vi "wathc for sweep files.vi"() -> ()   [LabVIEW 2010]
uses:
  watch for sweep file.ctl
panel:
  in  "watch for sweep files in":T1={"file path"=path "C:/data/RUS/Experiment/ProbeTest/systemtest/sweep1", "Watch for sweep files?"=FALSE}
  out "cursor position":dbl=-1.0
  out "history length (min)":dbl=20.0
  out "sweep files in the folder":i32=-1
  out "seconds":i32=189
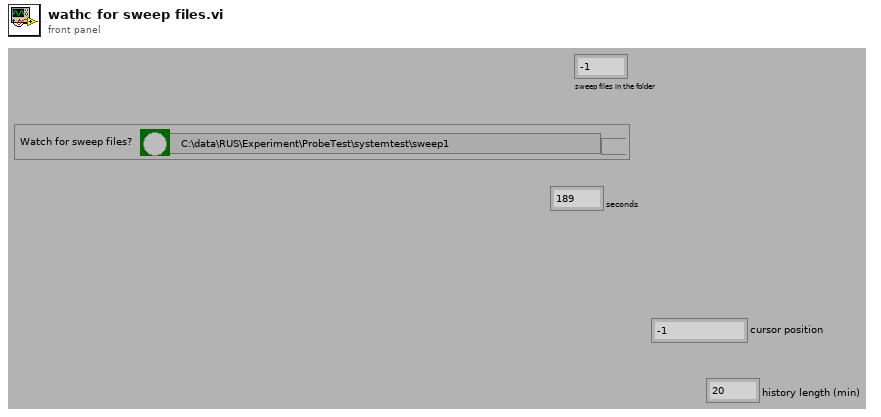
[diagram p1: front panel]
types:
  T1 = typedef "watch for sweep file.ctl" = cluster{"file path":path, "Watch for sweep files?":bool}
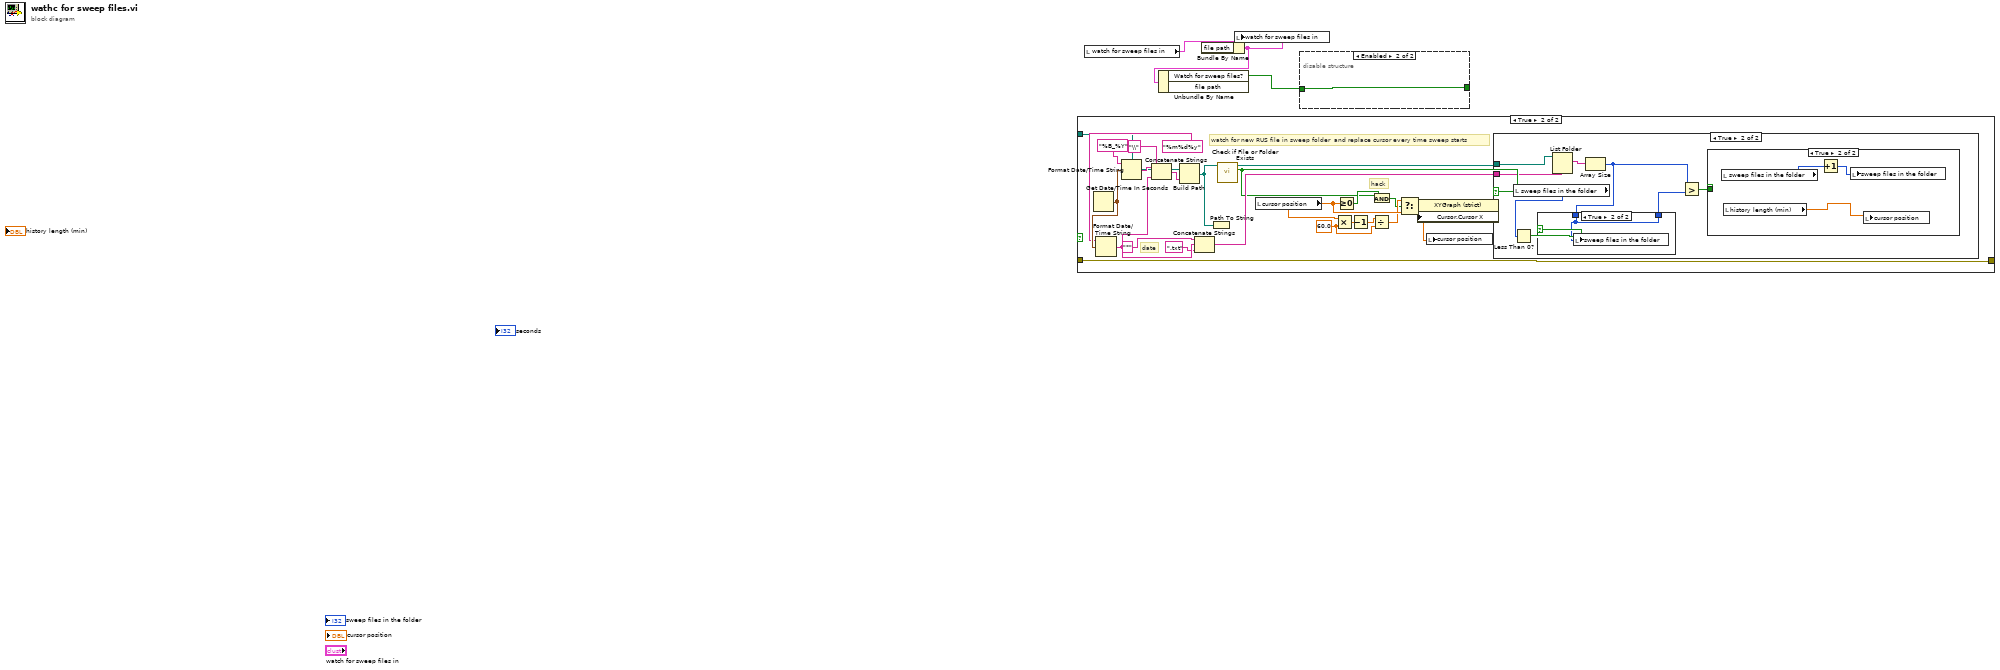
[diagram p0: block diagram]
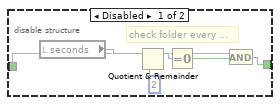
[diagram p2: hidden frame]
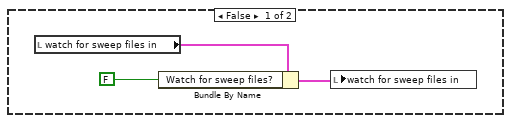
[diagram p4: hidden frame]
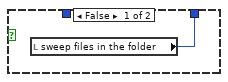
[diagram p6: hidden frame]
diagram:
  n1 = case shown="True" w5 {
    tunnel: [_ w18] -> w2
    tunnel: _ -> [w7 w8]
    tunnel: [w7 w8] -> _
    frame False {
    }
    frame True {
      w17 = 60.0 ("y")
      # "hack"
      # "watch for new RUS file in sweep folder  and replace cursor every time sweep starts"
      # "date"
      n2 = Get Date/Time In Seconds() -> (seconds since 1Jan1904=w27:timestamp)
      n3 = Format Date/Time String(time format string (%c)="%m%d%y", seconds (now)=w27) -> (date/time string=w23:string)  [unwired: 1 in]
      n4 = Format Date/Time String(time format string (%c)="%B_%Y", seconds (now)=w27) -> (date/time string=w29:string)  [unwired: 1 in]
      n5 = Concatenate Strings(w29, "\\" ("time format string (%c)"), w23) -> (w30:string)
      n6 = Build Path(base path=w18, name or relative path=w30) -> (appended path=w20:path)
      n7 = Concatenate Strings("*" ("time format string (%c)"), w23, ".txt" ("time format string (%c)")) -> (w21:string)
      n8 = Path To String(path=w20) -> ()  [unwired: 1 out]
      n9 = call <vilib>:"Check if File or Folder Exists.vi"("path"=w20) -> ("file or folder exists?"=w10:bool, "dup path"=w19:path)  [unwired: 8 in, 1 out]
      n10 = local read "cursor position"() -> (w14:dbl)
      n11 = Multiply(x=w14, y=w17) -> (x*y=w15:dbl)
      n12 = Greater Or Equal To 0?(x=w14) -> (x >= 0?=w12:bool)
      n13 = Decrement(x=w15) -> (x-1=w16:dbl)
      n14 = Divide(x=w16, y=w17) -> (x/y=w13:dbl)
      n15 = And(x=w10, y=w12) -> (x .and. y?=w11:bool)
      n16 = Select(t=w13, s=w11, f=w14) -> (s? t:f=w9:dbl)
      n17 = property on="Property Node" class="XYGraph (strict)"("Cursor.Cursor X"=w9) -> ()  [unwired: 2 in, 2 out]
      n18 = local write "cursor position"(w9) -> ()
      n19 = case shown="True" w10 {
        tunnel: w21 -> [_ w41]
        tunnel: w19 -> [_ w39]
        frame False {
          n20 = local read "watch for sweep files in"() -> (w33:T1)
          n21 = Bundle By Name(cluster=w33, "Watch for sweep files?"=FALSE) -> (w31:T1)
          n22 = local write "watch for sweep files in"(w31) -> ()
        }
        frame True {
          n23 = local read "sweep files in the folder"() -> (w36:i32)
          n24 = Less Than 0?(x=w36) -> (x < 0?=w35:bool)
          n25 = List Folder(path=w39, pattern=w41) -> (filenames=w40:string[])  [unwired: 2 in, 3 out]
          n26 = Array Size(array=w40) -> (size(s)=w38:i32)
          n27 = case shown="True" w35 {
            tunnel: w38 -> [_ w46]
            tunnel: [w45 w46] -> w37
            frame False {
              n28 = local read "sweep files in the folder"() -> (w45:i32)
            }
            frame True {
              n29 = local write "sweep files in the folder"(w46) -> ()
            }
          }
          n30 = Greater?(x=w38, y=w37) -> (0:w34:bool)
          n31 = case shown="True" w34 {
            tunnel: w34 -> [_ _]
            frame False {
            }
            frame True {
              n32 = local read "sweep files in the folder"() -> (w44:i32)
              n33 = local read "history length (min)"() -> (w42:dbl)
              n34 = Increment(x=w44) -> (x+1=w43:i32)
              n35 = local write "sweep files in the folder"(w43) -> ()
              n36 = local write "cursor position"(w42) -> ()
            }
          }
        }
      }
    }
  }
  n37 = local read "watch for sweep files in"() -> (w3:T1)
  n38 = Bundle By Name(cluster=w3) -> (w1:T1)  [unwired: 1 in]
  n39 = Unbundle By Name(w1) -> ("Watch for sweep files?"=w6:bool)  [unwired: 1 out]
  n40 = local write "watch for sweep files in"(w1) -> ()
  n41 = disable-structure shown="Enabled" {
    disable-tunnel: w6 -> [w48 w53]
    disable-tunnel: [w47 w53] -> w4
    frame Disabled {
      # "check folder every ..."
      n42 = local read "seconds"() -> (w49:i32)
      n43 = Quotient & Remainder(x=w49, y=2) -> (x-y*floor(x/y)=w51:i32)  [unwired: 1 out]
      n44 = Equal To 0?(x=w51) -> (x = 0?=w50:bool)
      n45 = And(x=w48, y=w50) -> (x .and. y?=w47:bool)
    }
    frame Enabled {
    }
  }
